vi "WPI_I2COpen.vi"(8 "error in":errorcluster, 9 "Device Address":u8, 10 "I2C Bus":T1=enum."Invalid") -> (0 "error out":errorcluster, 3 "I2CDevRef":T2={"DevStatus"={"status"=FALSE, "code"=0, "source"=""}, "Device Address"=0, "Handle"=0, "I2C Bus"=enum."Invalid"} {"Device Address" format="%.0x"})   [LabVIEW 2017]
doc: "Opens a reference to the I2C sensor you specify. You must open a reference before using any other VIs on this palette. After you open a reference to an I2C sensor, you can use the other I2C VIs to access and monitor the sensor.\n\nThis software is licensed. Open the labview\\readme\\WPI Robotics Library Open Source License.txt file for more information."
uses:
  <vilib>/Rock Robotics/WPI/I2C/WPI_I2CDevRef.ctl
  <vilib>/Rock Robotics/SystemInterfaces/i2clib/i2c_bus.ctl
  <vilib>/Rock Robotics/WPI/SPI/WPI_SPIBusCacheOp.ctl
  <vilib>/Rock Robotics/SystemInterfaces/NetworkCommunication/NetComm_UsageReport_ResourceType.ctl
  <vilib>/Rock Robotics/SystemInterfaces/System/FPGA_SystemGet.vi
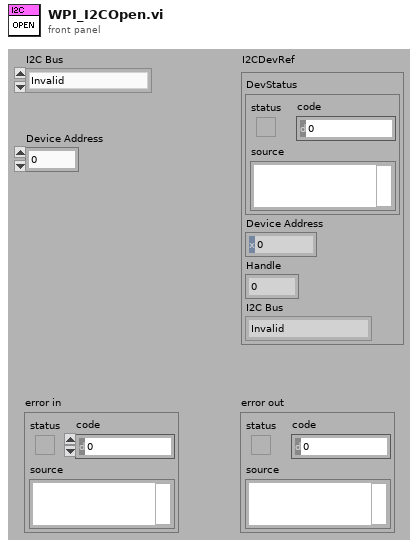
[diagram p1: front panel]
types:
  T1 = typedef "i2c_bus.ctl" = enum16{"I2C On-Board", "I2C MXP", "Invalid"}
  T2 = typedef "WPI_I2CDevRef.ctl" = cluster{"DevStatus":errorcluster, "Device Address":u8, "Handle":i32, "I2C Bus":T1}
  T3 = typedef "WPI_SPIBusCacheOp.ctl" = enum16{"Acquire", "Release", "Status"}
  T4 = typedef "NetComm_UsageReport_ResourceType.ctl" = enum8{"Controller", "Module", "Language", "CANPlugin", "Accelerometer", "ADXL345", "AnalogChannel", "AnalogTrigger", "AnalogTriggerOutput", "CANJaguar", "Compressor", "Counter", "Dashboard", "DigitalInput", "DigitalOutput", "DriverStationCIO", "DriverStationEIO", "DriverStationLCD", "Encoder", "GearTooth", "Gyro", "I2C", "Framework", "Jaguar", "Joystick", "Kinect", "KinectStick", "PIDController", "Preferences", "PWM", "Relay", "RobotDrive", "SerialPort", "Servo", "Solenoid", "SPI", "Task", "Ultrasonic", "Victor", "Button", "Command", "AxisCamera", "PCVideoServer", "SmartDashboard", "Talon", "HiTechnicColorSensor", "HiTechnicAccel", "HiTechnicCompass", "SRF08", "AnalogOutput", "Victor SP", "Talon SRX", "CAN Talon SRX", "ADXL362 Accel", "ADXRS450 Gyro", "Rev SPARK", "Mindsensors SD540", "Digital Filter", "ADIS16448", "PDP", "PCM", "PigeonIMU", "Nidec Brushless", "CTRE CANifier", "CTRE Future 0", "CTRE Future 1", "CTRE Future 2", "CTRE Future 3", "CTRE Future 4", "CTRE Future 5", "CTRE Future 6"}
  T5 = typedef "FPGA_DIODevRef.ctl" = cluster{"DevStatus":errorcluster}
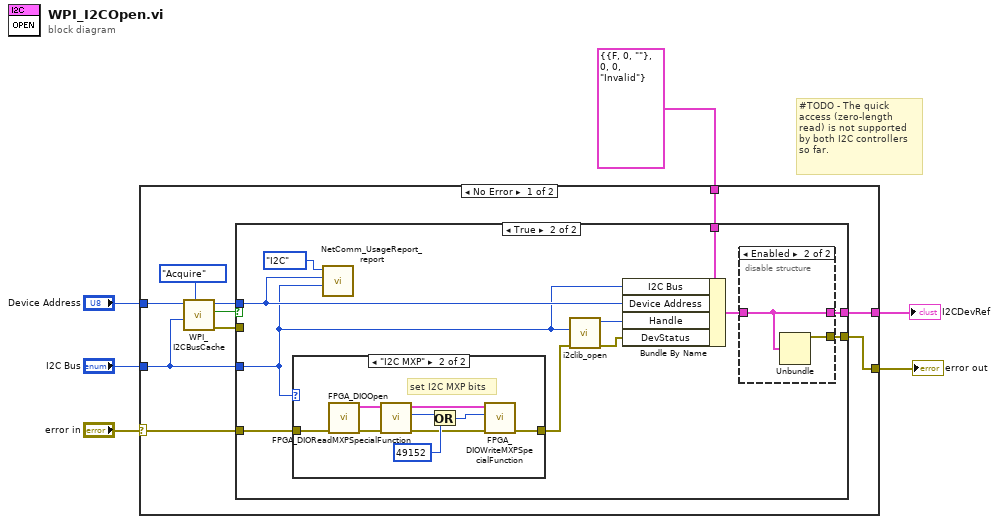
[diagram p0: block diagram]
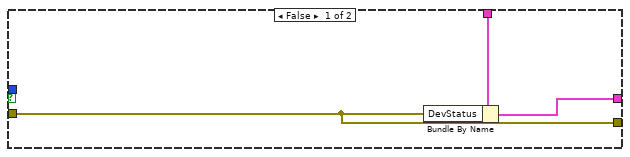
[diagram p2: hidden frame]
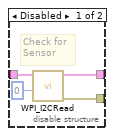
[diagram p4: hidden frame]
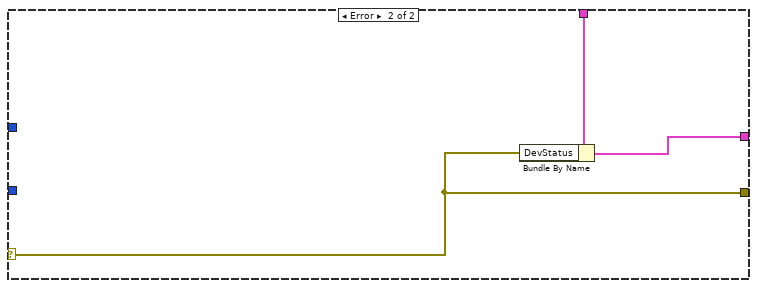
[diagram p5: hidden frame]
diagram:
  # "#TODO - The quick access (zero-length read) is not supported by both I2C controllers so far."
  n1 = case shown="No Error" "error in" {
    selector: "error in" -> [w14 w47]
    tunnel: T2 {"DevStatus"={"status"=FALSE, "code"=0, "source"=""}, "Device Address"=0, "Handle"=0, "I2C Bus"=enum."Invalid"} ("DigitalInputDevRef") -> [w15 w49]
    tunnel: [w11 w48] -> w4
    tunnel: [w16 w47] -> w3
    tunnel: "Device Address" -> [w9 _]
    tunnel: "I2C Bus" -> [w10 _]
    frame No Error {
      n2 = call <vilib>:"WPI_I2CBusCache.vi"("Operation"=WPI_SPIBusCacheOp."Acquire", "I2C Bus"=w10, "Device Address"=w9) -> ("error out"=w7:errorcluster, "Allocated?"=w8:bool, "Device Address Allocated"=w13:u8)  [unwired: 6 in]
      n3 = case shown="True" w8 {
        tunnel: [w17 w29] -> w16
        tunnel: w15 -> [w19 w24]
        tunnel: w10 -> [_ w20]
        tunnel: w14 -> [_ w23]
        tunnel: w13 -> [_ w21]
        tunnel: [w18 w28] -> w11
        tunnel: w7 -> [w17 _]
        frame False {
          n4 = Bundle By Name(cluster=w19, "DevStatus"=w17) -> (w18:T2)
        }
        frame True {
          n5 = case shown="\"I2C MXP\"" w20 {
            tunnel: w23 -> [w31 w40]
            tunnel: [w31 w39] -> w22
            frame "I2C On-Board", Default {
            }
            frame "I2C MXP" {
              # "set I2C MXP bits"
              n6 = call <vilib>:"FPGA_DIOOpen.vi"("error in (no error)"=w40) -> ("error out"=w37:errorcluster, "DIODeviceRef"=w38:T5)  [unwired: 1 in, 8 out]
              n7 = call <vilib>:"FPGA_DIOReadMXPSpecialFunction.vi"("error in (no error)"=w37, "DIODeviceRef In"=w38) -> ("error out"=w32:errorcluster, "EnableSpecialFunction"=w35:u16, "DIODeviceRef Out"=w36:T5)  [unwired: 7 in]
              n8 = Or(x=w35, y=u16 49152 ("EnableSpecialFunction")) -> (x .or. y?=w33:u16)
              n9 = call <vilib>:"FPGA_DIOWriteMXPSpecialFunction.vi"("error in (no error)"=w32, "EnableSpecialFunction"=w33, "DIODeviceRef In"=w36) -> ("error out"=w39:errorcluster)  [unwired: 7 in, 1 out]
            }
          }
          n10 = call <vilib>:"NetComm_UsageReport_report.vi"("Context"=w20, "Instance Number"=w21, "Resource Type"=NetComm_UsageReport_ResourceType."I2C") -> ()  [unwired: 9 in]
          n11 = call <vilib>:"i2clib_open.vi"("error in (no error)"=w22, "I2C Bus"=w20) -> ("error out"=w25:errorcluster, "I2C Reference Out"=w26:i32)  [unwired: 8 in]
          n12 = Bundle By Name(cluster=w24, "I2C Bus"=w20, "Device Address"=w21, "Handle"=w26, "DevStatus"=w25) -> (w30:T2)
          n13 = disable-structure shown="Enabled" {
            disable-tunnel: w30 -> [w44 w46]
            disable-tunnel: [w43 w45] -> w29
            disable-tunnel: [w42 w46] -> w28
            frame Disabled {
              # "Check for\nSensor"
              n14 = call <vilib>:"WPI_I2CRead.vi"("I2CBytesToRead"=u8 0, "I2CDevRef"=w44) -> ("error out"=w43:errorcluster, "I2CDevRef"=w42:T2)  [unwired: 2 in, 6 out]
            }
            frame Enabled {
              n15 = Unbundle(w46) -> ("DevStatus"=w45:errorcluster)  [unwired: 3 out]
            }
          }
        }
      }
    }
    frame Error {
      n16 = Bundle By Name(cluster=w49, "DevStatus"=w47) -> (w48:T2)
    }
  }
  "I2CDevRef" <- w4
  "error out" <- w3
